vi "Write key.vi"(8 "error in (no error)":errorcluster, 10 "key":string, 11 "Update CVT CMD in":refnum<class "Update CVT CMD.lvclass">) -> (0 "error out":errorcluster, 3 "Update CVT CMD out":refnum<class "Update CVT CMD.lvclass">)   [LabVIEW 2014, in "Update CVT CMD.lvclass"]
uses:
  Update CVT CMD.lvclass
  Update CVT CMD.lvclass/Update CVT CMD.ctl
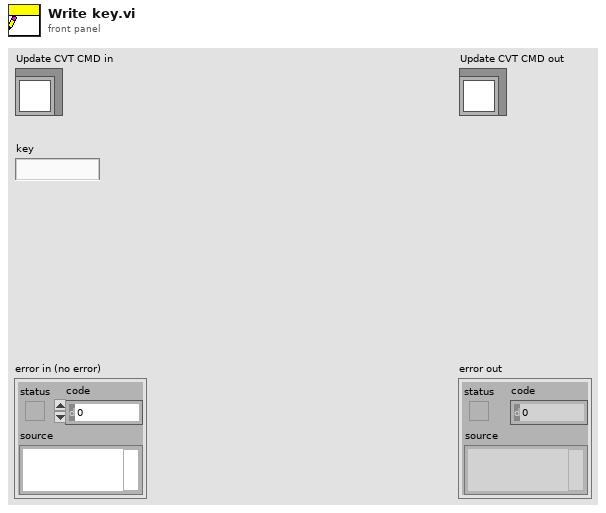
[diagram p1: front panel]
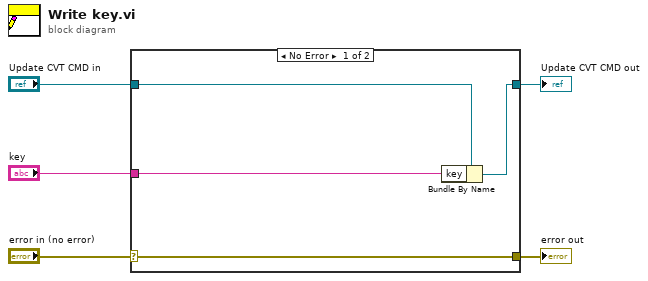
[diagram p0: block diagram]
diagram:
  n1 = case shown="No Error" "error in (no error)" {
    selector: "error in (no error)" -> [w9 w10]
    tunnel: [w9 w10] -> w4
    tunnel: [w7 w11] -> w2
    tunnel: "Update CVT CMD in" -> [w8 w11]
    tunnel: "key" -> [w6 _]
    frame No Error {
      n2 = Bundle By Name(cluster=w8, "key"=w6) -> (w7:refnum<class "Update CVT CMD.lvclass">)
    }
    frame Error {
    }
  }
  "error out" <- w4
  "Update CVT CMD out" <- w2
